vi "GlobalCurrentFrame.vi"() -> ()   [LabVIEW 2010]
panel:
  in  "Current Frame":u32
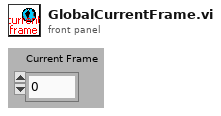
[diagram p1: front panel]
diagram:
